vi "FloatToString (SubVI).vi"(11 "Numeric":sgl) -> (3 "String":string)   [LabVIEW 2017, in "LV_Unicorn.lvlib"]
uses:
  LV_Unicorn.lvlib
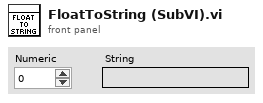
[diagram p1: front panel]
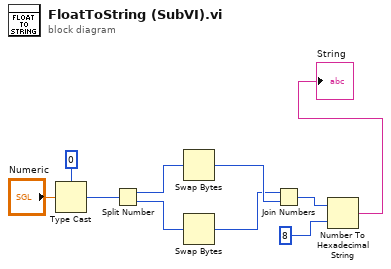
[diagram p0: block diagram]
diagram:
  n1 = Type Cast(type=u32 0 ("(hi.lo)"), x="Numeric") -> (*(type *) &x=w2:u32)
  n2 = Split Number(x=w2) -> (hi(x)=w3:u16, lo(x)=w4:u16)
  n3 = Swap Bytes(anything=w3) -> (byte swapped=w6:u16)
  n4 = Swap Bytes(anything=w4) -> (byte swapped=w5:u16)
  n5 = Join Numbers(hi=w5, lo=w6) -> ((hi.lo)=w7:u32)
  n6 = Number To Hexadecimal String(1:i16 8 ("width (-)"), 2:w7) -> (0:→"String":string)
